vi "VariableValueToString.vi"(5 "SignificantDigits (8)":u32=8, 7 "Format (SI notation)":T1(ring)=enum."SI notation", 11 "VariableValue":refnum<class "VariableValue.lvclass">) -> (3 "VariableValueString":string)   [LabVIEW 2013, in "VariableManagerAPI.lvlib"]
uses:
  VariableManagerAPI.lvlib
  VariableValue/VariableValue.lvclass
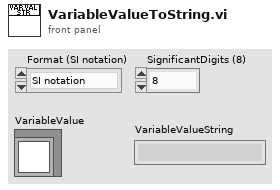
[diagram p1: front panel]
types:
  T1 = enum16{"Floating point", "Scientific SI", "Automatic SI", "SI notation"}
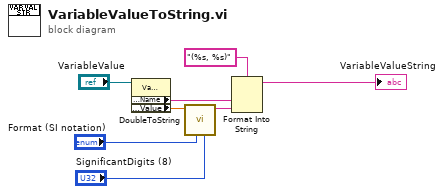
[diagram p0: block diagram]
diagram:
  n1 = property class="VariableValue.lvclass"(reference="VariableValue") -> ("Accessors:Name"=w7:string, "Accessors:Value"=w4:dbl)  [unwired: 1 in, 2 out]
  n2 = call "DoubleToString.vi"("SignificantDigits (8)"="SignificantDigits (8)", "Format (SI notation)"="Format (SI notation)", "Double"=w4) -> ("String"=w3:string)  [unwired: 8 in]
  n3 = Format Into String(format string="(%s, %s)", w7, w3) -> (resulting string=→"VariableValueString":string)  [unwired: 2 in, 1 out]
